vi "Send_SMS.vi"(0 "Mobile Number and code":string) -> (1 "Send?":bool, 2 "Mobile Number":string, 3 "Send Code":u32)   [LabVIEW 2010]
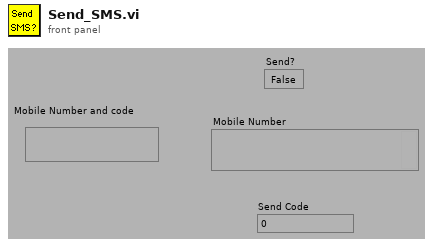
[diagram p1: front panel]
types:
  T1 = cluster{"second":i32, "minute":i32, "hour":i32, "day of month":i32, "month":i32, "year":i32, "day of week":i32, "day of year":i32, "is DST":i32}
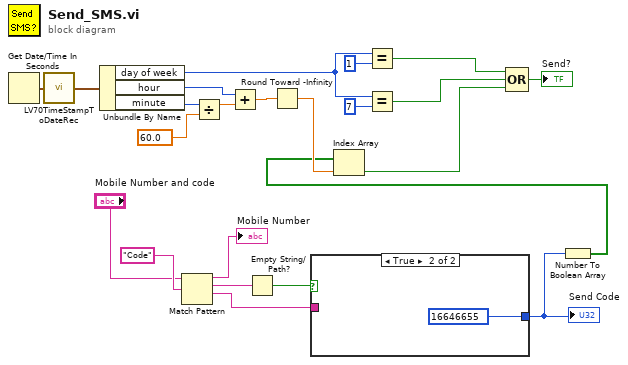
[diagram p0: block diagram]
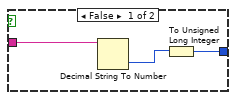
[diagram p2: hidden frame]
diagram:
  n1 = Get Date/Time In Seconds() -> (seconds since 1Jan1904=w1:timestamp)
  n2 = call <vilib>:"LV70TimeStampToDateRec.vi"("time stamp"=w1) -> ("date time rec"=w23:T1)
  n3 = Unbundle By Name(w23) -> ("day of week"=w20:i32, "hour"=w15:i32, "minute"=w17:i32)
  n4 = Match Pattern(string="Mobile Number and code", regular expression="Code" ("String to match")) -> (before substring=→"Mobile Number":string, match substring=w6:string, after substring=w4:string)  [unwired: 2 out]
  n5 = Divide(x=w17, y=60.0) -> (x/y=w14:dbl)
  n6 = Add(x=w15, y=w14) -> (x+y=w12:dbl)
  n7 = Empty String/Path?(string/path=w6) -> (empty?=w5:bool)
  n8 = Round Toward -Infinity(1:w12) -> (0:w10:dbl)
  n9 = case shown="True" w5 {
    tunnel: w4 -> [w26 _]
    tunnel: [w24 u32 16646655 ("number")] -> w3
    frame False {
      n10 = Decimal String To Number(string=w26) -> (number=w25:i32)  [unwired: 3 out]
      n11 = To Unsigned Long Integer(number=w25) -> (unsigned 32bit integer=w24:u32)
    }
    frame True {
    }
  }
  "Send Code" <- w3
  n12 = Equal?(x=w20, y=1) -> (x = y?=w19:bool)
  n13 = Equal?(x=w20, y=7) -> (x = y?=w18:bool)
  n14 = Number To Boolean Array(number=w3) -> (Boolean array=w2:bool[])
  n15 = Index Array(array=w2, index=w10) -> (element=w11:bool)
  n16 = Compound Arithmetic op=OR(w19, w18, w11) -> (→"Send?":bool)
